vi "H5Read Dataspace Helper.vi"(5 "HDF5 Memory Space":T1, 6 "Old Data":variant, 7 "TD Enum":T2 format="%.0x", 8 "error out":errorcluster, 11 "New Data":variant) -> (0 "error":errorcluster, 3 "Data out":variant)   [LabVIEW 2017]
uses:
  <userlib>/_OpenG.lib/lvdata/lvdata.llb/Type Descriptor Enumeration__ogtk.ctl
  <vilib>/UPVI/lvhdf5/library.llb/HDF5 Ref.ctl
  <vilib>/UPVI/lvhdf5/dataspace.llb/H5S_sel_type.ctl
panel:
  # "LVHDF5 Toolkit\nCopyright (c) 2005-2013 by Jason D. Sommerville\nCopyright (c) 2014 by UPVI, LLC.\n\nThis use and distribution of this file is governed by the terms found in \nLICENSE.txt distributed with this toolkit and installed at\n <user.lib>\\_lvhdf5\\LICENSE.txt"
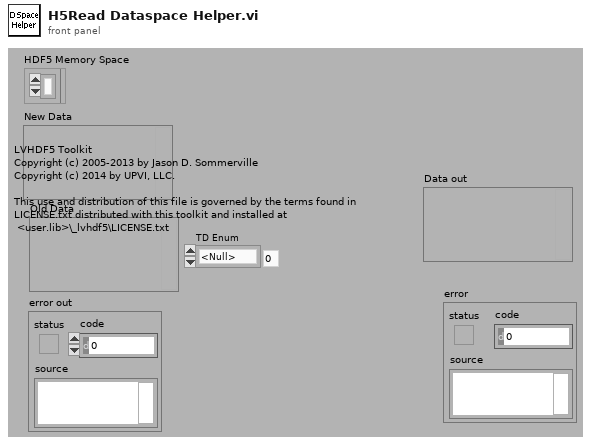
[diagram p1: front panel]
types:
  T1 = typedef "HDF5 Ref.ctl" = refnum<k1>
  T2 = typedef "Type Descriptor Enumeration__ogtk.ctl" = enum8{"<Null>", "I8", "I16", "I32", "I64", "U8", "U16", "U32", "U64", "SGL", "DBL", "EXT", "CSG", "CDB", "CXT", "0x0F", "0x10", "0x11", "0x12", "0x13", "0x14", "Enum U8", "Enum U16", "Enum U32", "Enum U64", "SGL PQ", "DBL PQ", "EXT PQ", "CSG PQ", "CDB PQ", "CXT PQ", "0x1F", "0x20", "Boolean", "0x22", "0x23", "0x24", "0x25", "0x26", "0x27", "0x28", "0x29", "0x2A", "0x2B", "0x2C", "0x2D", "0x2E", "0x2F", "String", "0x31", "Path", "Pict", "0x34", "0x35", "0x36", "DAQ", "0x38", "0x39", "0x3A", "0x3B", "0x3C", "0x3D", "0x3E", "0x3F", "Array", "0x41", "0x42", "0x43", "0x44", "0x45", "0x46", "0x47", "0x48", "0x49", "0x4A", "0x4B", "0x4C", "0x4D", "0x4E", "0x4F", "Cluster", "0x51", "0x52", "Variant", "Waveform", "0x55", "0x56", "0x57", "0x58", "0x59", "0x5A", "0x5B", "0x5C", "0x5D", "0x5E", "0x5F", "0x60", "0x61", "0x62", "0x63", "0x64", "0x65", "0x66", "0x67", "0x68", "0x69", "0x6A", "0x6B", "0x6C", "0x6D", "0x6E", "0x6F", "Refnum"}
  T3 = typedef "H5S_sel_type.ctl" = i32
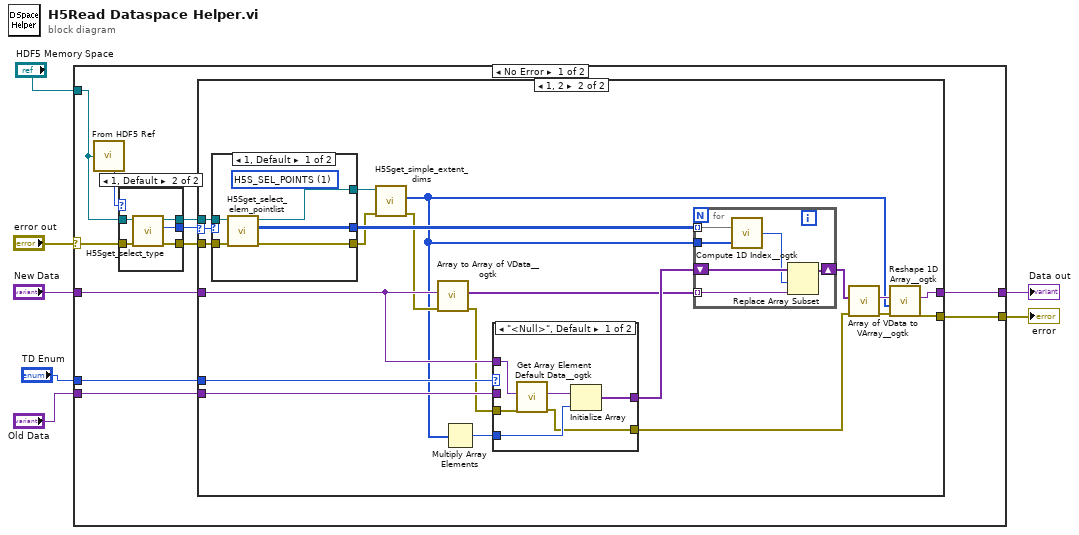
[diagram p0: block diagram]
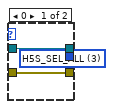
[diagram p2: hidden frame]
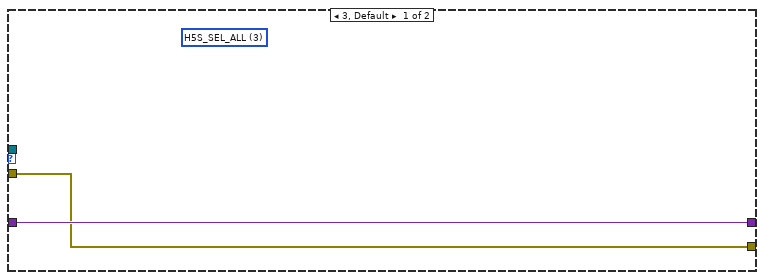
[diagram p3: hidden frame]
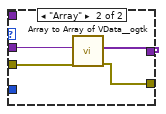
[diagram p4: hidden frame]
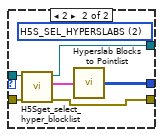
[diagram p5: hidden frame]
diagram:
  n1 = case shown="No Error" "error out" {
    selector: "error out" -> [w18 w78]
    tunnel: "New Data" -> [w13 w77]
    tunnel: "HDF5 Memory Space" -> [w10 _]
    tunnel: [w14 w77] -> w4
    tunnel: [w12 w78] -> w5
    tunnel: "Old Data" -> [w11 _]
    tunnel: "TD Enum" -> [w8 _]
    frame No Error {
      n2 = call <vilib>:"From HDF5 Ref.vi"("HDF5 Ref"=w10) -> ("I32"=w9:i32)
      n3 = case shown="1, Default" w9 {
        tunnel: w18 -> [w20 w26]
        tunnel: w10 -> [w19 w25]
        tunnel: [w19 w24] -> w17
        tunnel: [w20 w23] -> w16
        tunnel: [w21 w22] -> w15
        frame 0 {
          w21 = T3 3 items=["H5S_SEL_ERROR"=-1, "H5S_SEL_NONE"=0, "H5S_SEL_POINTS"=1, "H5S_SEL_HYPERSLABS"=2, "H5S_SEL_ALL"=3] ("Selection type")
        }
        frame 1, Default {
          n4 = call <vilib>:"H5Sget_select_type.vi"("error in (no error)"=w26, "HDF5 Dataspace Ref"=w25) -> ("error out"=w23:errorcluster, "Selection type"=w22:T3, "HDF5 Ref out"=w24:T1)  [unwired: 5 in]
        }
      }
      n5 = case shown="1, 2" w15 {
        selector: w15 -> [_ w47]
        tunnel: w17 -> [_ w49]
        tunnel: w16 -> [w27 w48]
        tunnel: [w28 w31] -> w14
        tunnel: w13 -> [w28 w39]
        tunnel: [w27 w29] -> w12
        tunnel: w11 -> [_ w45]
        tunnel: w8 -> [_ w46]
        frame 3, Default {
          (unwired) T3 3 items=["H5S_SEL_ERROR"=-1, "H5S_SEL_NONE"=0, "H5S_SEL_POINTS"=1, "H5S_SEL_HYPERSLABS"=2, "H5S_SEL_ALL"=3] ("Selection type")
        }
        frame 1, 2 {
          n6 = case shown="1, Default" w47 {
            tunnel: w49 -> [w69 w75]
            tunnel: w48 -> [w70 w76]
            tunnel: [w68 w73] -> w43
            tunnel: [w67 w71] -> w41
            tunnel: [w66 w72] -> w40
            frame 1, Default {
              (unwired) T3 1 items=["H5S_SEL_ERROR"=-1, "H5S_SEL_NONE"=0, "H5S_SEL_POINTS"=1, "H5S_SEL_HYPERSLABS"=2, "H5S_SEL_ALL"=3] ("Selection type")
              n7 = call <vilib>:"H5Sget_select_elem_pointlist.vi"("error in (no error)"=w70, "HDF5 Space Ref"=w69) -> ("error out"=w66:errorcluster, "Pointlist"=w68:u64[][], "HDF5 Ref out"=w67:T1)  [unwired: 5 in]
            }
            frame 2 {
              (unwired) T3 2 items=["H5S_SEL_ERROR"=-1, "H5S_SEL_NONE"=0, "H5S_SEL_POINTS"=1, "H5S_SEL_HYPERSLABS"=2, "H5S_SEL_ALL"=3] ("Selection type")
              n8 = call <vilib>:"H5Sget_select_hyper_blocklist.vi"("error in (no error)"=w76, "HDF5 Space Ref"=w75) -> ("error out"=w72:errorcluster, "Hyperslab Blocks"=w74:cluster{"Start":u64[], "Opposite":u64[]}[], "HDF5 Ref out"=w71:T1)  [unwired: 5 in]
              n9 = call <vilib>:"Hyperslab Blocks to Pointlist.vi"("Hyperslab Blocks"=w74) -> ("Pointlist"=w73:u64[][])
            }
          }
          n10 = call <vilib>:"H5Sget_simple_extent_dims.vi"("error in (no error)"=w40, "HDF5 Space Ref"=w41) -> ("error out"=w38:errorcluster, "Dims"=w33:u64[])  [unwired: 4 in, 2 out]
          n11 = call <userlib>:"Array to Array of VData__ogtk.vi"("error in (no error)"=w38, "MultiD Array"=w39) -> ("error out"=w34:errorcluster, "1D Array of Variants"=w37:variant[])  [unwired: 8 in]
          n12 = Multiply Array Elements(1:w33) -> (0:w42:u64)
          n13 = case shown="\"<Null>\", Default" w46 {
            tunnel: [w51 w58] -> w44
            tunnel: w45 -> [_ w59]
            tunnel: w42 -> [w55 _]
            tunnel: w39 -> [w50 _]
            tunnel: w34 -> [w53 w57]
            tunnel: [w52 w56] -> w30
            frame "<Null>", Default {
              n14 = call <userlib>:"Get Array Element Default Data__ogtk.vi"("error in (no error)"=w53, "Array"=w50) -> ("error out"=w52:errorcluster, "Array Element Default Data"=w54:variant)  [unwired: 8 in]
              n15 = Initialize Array(w54, w55) -> (w51:variant[])
            }
            frame "Array" {
              n16 = call <userlib>:"Array to Array of VData__ogtk.vi"("error in (no error)"=w57, "MultiD Array"=w59) -> ("error out"=w56:errorcluster, "1D Array of Variants"=w58:variant[])  [unwired: 8 in]
            }
          }
          n17 = for {
            shift-right: [w60] -> w32
            shift-left: w44 -> [w63]
            tunnel: w43 -> [w65] mode=indexing
            tunnel: w33 -> [w64]
            tunnel: w37 -> [w62] mode=indexing
            n18 = call <userlib>:"Compute 1D Index__ogtk.vi"("Size(s)"=w64, "Indices"=w65) -> ("1D Index"=w61:i32)
            n19 = Replace Array Subset(array=w63, new element=w62, index=w61) -> (w60:variant[])
          }
          n20 = call <userlib>:"Array of VData to VArray__ogtk.vi"("error in (no error)"=w30, "1D Array of VData"=w32) -> ("error out"=w36:errorcluster, "VArray"=w35:variant)  [unwired: 8 in]
          n21 = call <userlib>:"Reshape 1D Array__ogtk.vi"("error in (no error)"=w36, "Size(s)"=w33, "1D Array"=w35) -> ("error out"=w29:errorcluster, "Reshaped VArray"=w31:variant)  [unwired: 7 in]
        }
      }
    }
    frame Error {
    }
  }
  "error" <- w5
  "Data out" <- w4
